vi "Select online Station.vi"(8 "error in (no error)":errorcluster, 10 "FP Frontmost":bool=TRUE, 11 "OPC Server in":refnum<class "OPC Server.lvclass">) -> (0 "error out":errorcluster, 3 "OPC Server out":refnum<class "OPC Server.lvclass">)   [LabVIEW 2021, in "OPC Server.lvlib" / "OPC Server.lvclass"]
uses:
  OPC Server.lvclass
  OPC Server.lvclass/OPC Server.ctl
  Station Panel/Panel Messages/FP Front most Msg/FP Front most Msg.lvclass/FP Front most Msg.ctl
  <vilib>/ActorFramework/Message Enqueuer/Message Enqueuer.lvclass/Message Enqueuer.ctl
  <vilib>/ActorFramework/Message Enqueuer/Enqueue.vi
  Station Panel/Panel Messages/FP Front most Msg/FP Front most Msg.lvclass
  C:/Program Files/National Instruments/LabVIEW 2021/vi.lib/ActorFramework/Message/Message.lvclass
  <vilib>/ActorFramework/Message Priority Queue/Priority Enqueue.vi
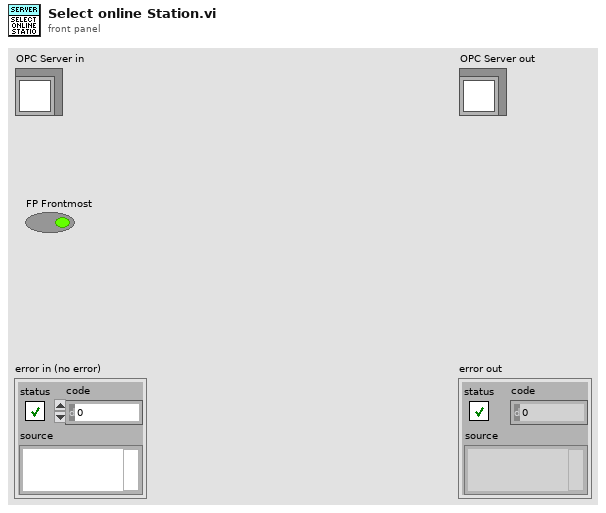
[diagram p1: front panel]
types:
  T1 = map{string, refnum<class "Message Enqueuer.lvclass">}
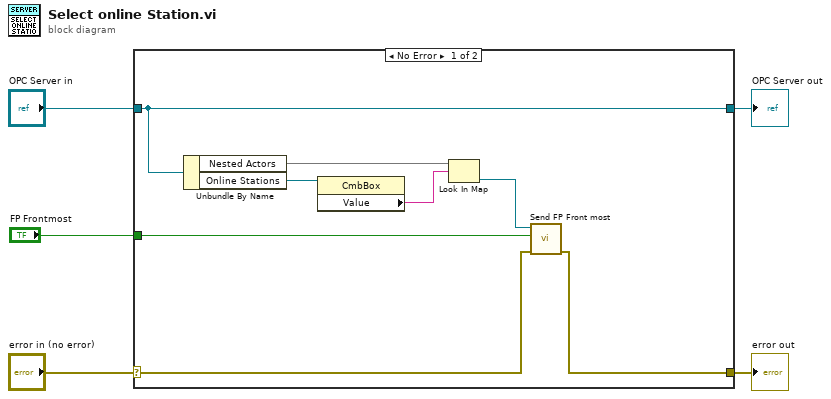
[diagram p0: block diagram]
diagram:
  n1 = case shown="No Error" "error in (no error)" {
    selector: "error in (no error)" -> [w13 w15]
    tunnel: [w6 w15] -> w4
    tunnel: [w7 w14] -> w2
    tunnel: "OPC Server in" -> [w7 w14]
    tunnel: "FP Frontmost" -> [w8 _]
    frame No Error {
      n2 = Unbundle By Name(w7) -> ("Nested Actors"=w12:T1, "Online Stations"=w11:refnum<vi>)
      n3 = property class="CmbBox"(reference=w11) -> ("Value"=w10:string)  [unwired: 1 in, 2 out]
      n4 = Look In Map(map=w12, key=w10) -> (value=w9:refnum<class "Message Enqueuer.lvclass">)  [unwired: 1 in, 1 out]
      n5 = call "Send FP Front most.vi"("error in (no error)"=w13, "FP Frontmost"=w8, "Message Enqueuer"=w9) -> ("error out"=w6:errorcluster)  [unwired: 7 in, 1 out]
    }
    frame Error {
    }
  }
  "error out" <- w4
  "OPC Server out" <- w2
